vi "Waveform Obj Class Test.vi"() -> ()   [LabVIEW 2020]
uses:
  Libraries/Waveform Obj Class/Sine Wave/Sine Wave.lvclass
  Libraries/Waveform Obj Class/Square Wave/Square Wave.lvclass
  Libraries/Waveform Obj Class/Waveform Gen/Waveform Gen.lvclass
  Libraries/Waveform Obj Class/Triangle Wave/Triangle Wave.lvclass
  Libraries/Waveform Obj Class/Sawtooth Wave/Sawtooth Wave.lvclass
  Libraries/Waveform Obj Class/Square Wave/Controls/Slope Type.ctl
  Libraries/Waveform Obj Class/Waveform Gen/Controls/repeat scale.ctl
panel:
  in  "repeat type":T1
  in  "slope type":T2=enum."Exp."
  in  "slope length":u32=25
  in  "Type":enum16{"Sine", "Square", "Triangle", "Sawtooth"}(ring)
  out "크기":i32
  out "웨이브폼 그래프":dbl[](graph)
  in  "amplitude":dbl=5.0
  in  "cycle":dbl=1.0
  in  "frequency":dbl=160.0
  in  "offset":dbl
  in  "phase":dbl
  in  "sampling rate":dbl=48000.0
  in  "scale":dbl=1.0
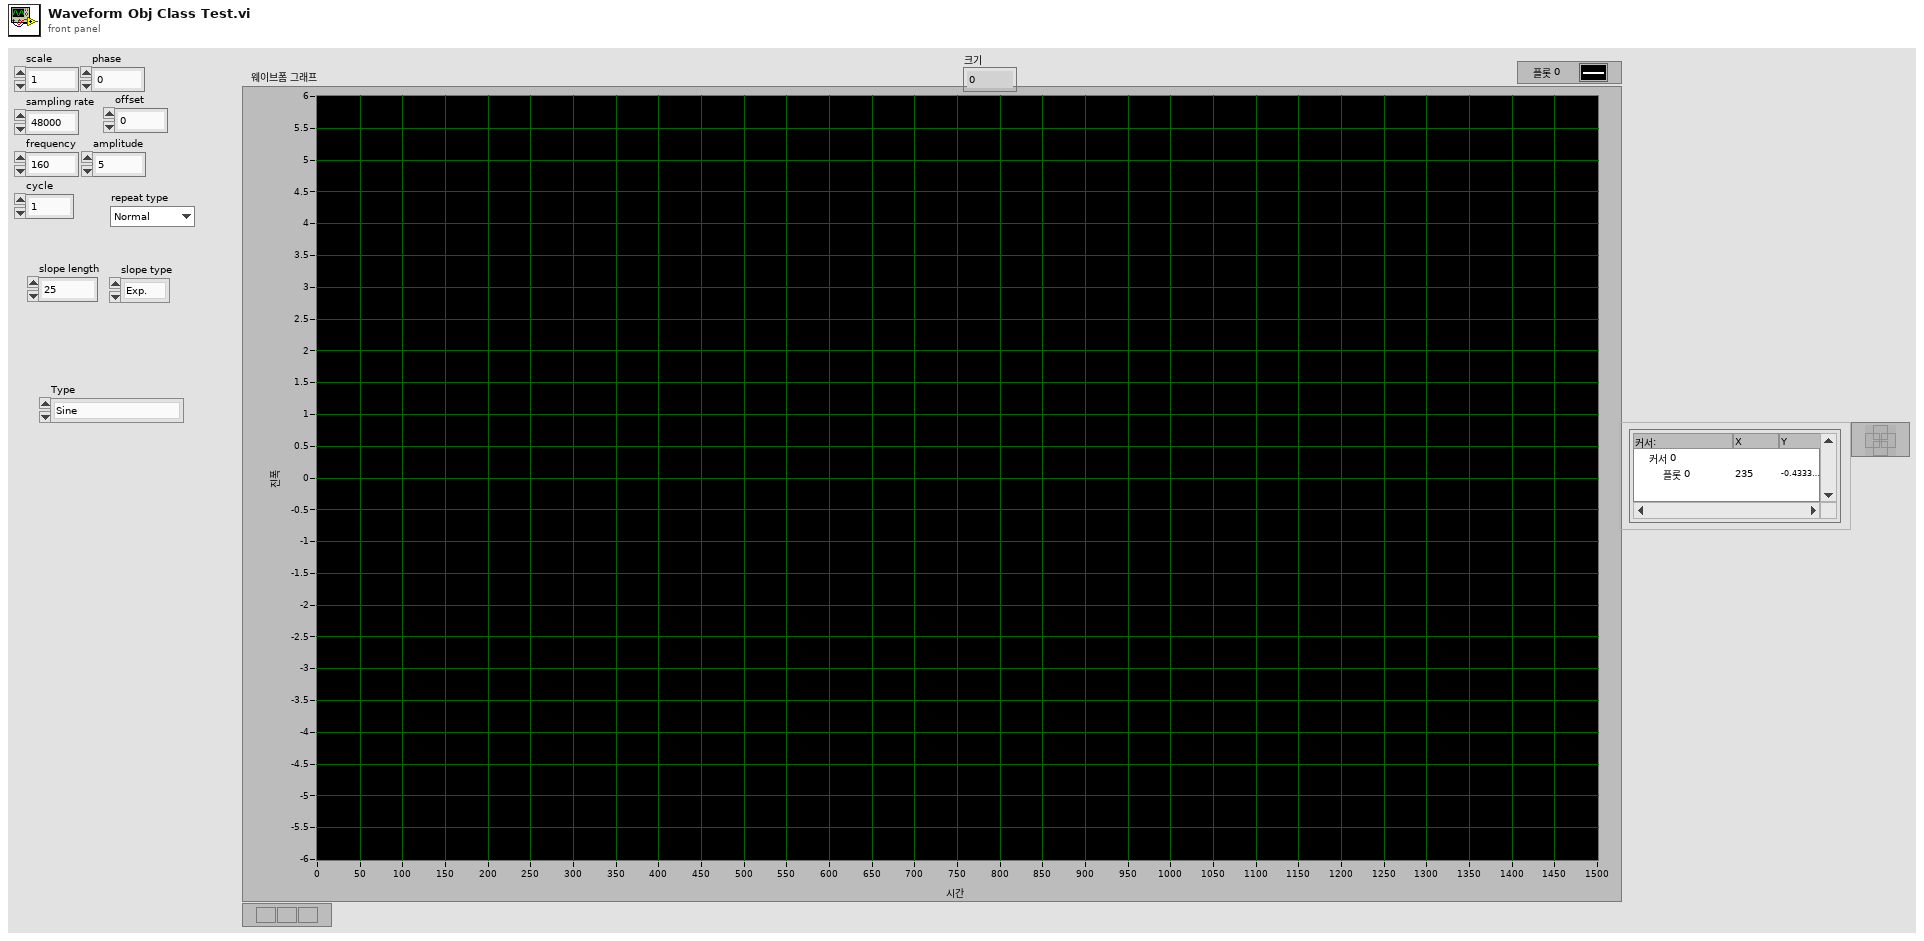
[diagram p1: front panel]
types:
  T1 = typedef "Waveform Gen.lvclass/repeat scale.ctl" = enum16{"Normal", "Lin. Up", "Lin. Down", "Exp. Up", "Exp. Down"}
  T2 = typedef "Square Wave.lvclass/Slope Type.ctl" = enum16{"None", "Lin.", "Exp."}
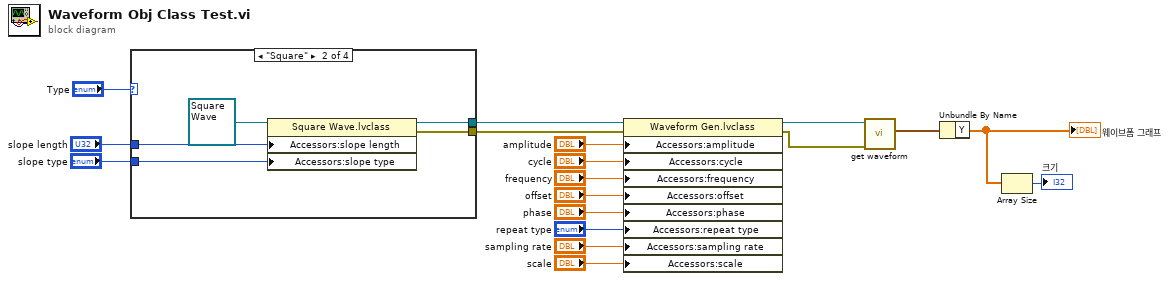
[diagram p0: block diagram]
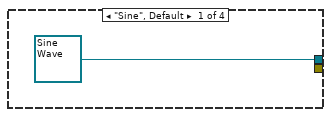
[diagram p2: hidden frame]
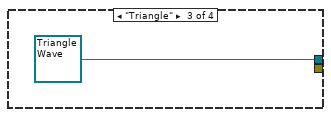
[diagram p3: hidden frame]
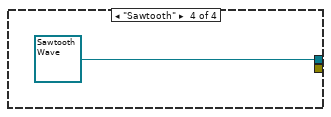
[diagram p4: hidden frame]
diagram:
  n1 = case shown="\"Square\"" "Type" {
    tunnel: [refnum<class "Sine Wave.lvclass"> refnum ("Sine Wave.lvclass") w23 refnum<class "Triangle Wave.lvclass"> refnum ("Triangle Wave.lvclass") refnum<class "Sawtooth Wave.lvclass"> refnum ("Sawtooth Wave.lvclass")] -> w9
    tunnel: "slope length" -> [_ w22 _ _]
    tunnel: "slope type" -> [_ w21 _ _]
    tunnel: [_ w20 _ _] -> w3
    frame "Sine", Default {
    }
    frame "Square" {
      n2 = property class="Square Wave.lvclass"(reference=refnum<class "Square Wave.lvclass"> refnum ("Square Wave.lvclass"), "Accessors:slope length"=w22, "Accessors:slope type"=w21) -> (reference out=w23:refnum<class "Square Wave.lvclass">, error out=w20:errorcluster)  [unwired: 1 in]
    }
    frame "Triangle" {
    }
    frame "Sawtooth" {
    }
  }
  n3 = property class="Waveform Gen.lvclass"(reference=w9, error in=w3, "Accessors:amplitude"="amplitude", "Accessors:cycle"="cycle", "Accessors:frequency"="frequency", "Accessors:offset"="offset", "Accessors:phase"="phase", "Accessors:repeat type"="repeat type", "Accessors:sampling rate"="sampling rate", "Accessors:scale"="scale") -> (reference out=w8:refnum<class "Waveform Gen.lvclass">, error out=w7:errorcluster)
  n4 = call-dynamic "get waveform.vi"("error in (no error)"=w7, "Waveform Obj 입력"=w8) -> ("waveform"=w2:waveform(dbl))  [unwired: 7 in, 2 out]
  n5 = Unbundle By Name(w2) -> ("Y"=w11:dbl[])
  "웨이브폼 그래프" <- w11
  n6 = Array Size(array=w11) -> (size(s)=→"크기":i32)
